vi "Export from Listbox to CSV.vi"(8 "error in (no error)":errorcluster, 10 "Name":string, 11 "MulticolumnListbox in":refnum<vi>) -> (0 "error out":errorcluster)   [LabVIEW 2019, in "Control Addon System Explorer.lvlib"]
uses:
  Control Addon System Explorer.lvlib
  Addon Shared/Control Addon Shared.lvlib
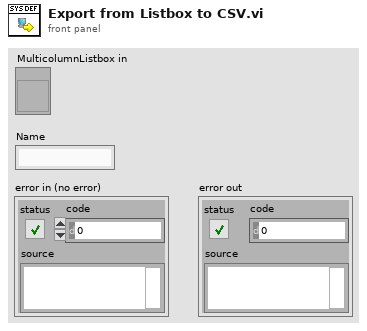
[diagram p1: front panel]
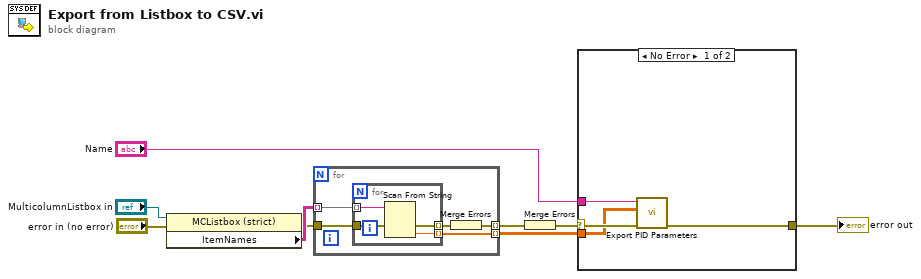
[diagram p0: block diagram]
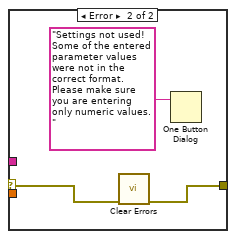
[diagram p2: hidden frame]
diagram:
  n1 = property class="MCListbox (strict)"(reference="MulticolumnListbox in", error in="error in (no error)") -> (error out=w5:errorcluster, "ItemNames"=w6:string[][])  [unwired: 1 out]
  n2 = for {
    tunnel: w6 -> [w14] mode=indexing
    tunnel: [w13] -> w1 mode=indexing
    tunnel: [w12] -> w9 mode=indexing
    tunnel: w5 -> [w10]
    n3 = for {
      tunnel: w14 -> [w18] mode=indexing
      tunnel: [w17] -> w13 mode=indexing
      tunnel: [w16] -> w11 mode=indexing
      tunnel: w10 -> [w15]
      n4 = Scan From String(input string=w18, error in=w15) -> (error out=w16:errorcluster, output 1=w17:dbl)  [unwired: 3 in, 2 out]
    }
    n5 = Merge Errors(w11) -> (w12:errorcluster)
  }
  n6 = Merge Errors(w9) -> (w4:errorcluster)
  n7 = case shown="No Error" w4 {
    selector: w4 -> [w22 w25]
    tunnel: [w21 w23] -> w3
    tunnel: "Name" -> [w20 _]
    tunnel: w1 -> [w19 _]
    frame No Error {
      n8 = call "Export PID Parameters.vi"("error in"=w22, "Parameters"=w19, "Control Loop"=w20) -> ("error out"=w21:errorcluster)  [unwired: 8 in]
    }
    frame Error {
      n9 = call <vilib>:"Clear Errors.vi"("error in (no error)"=w25) -> ("error out"=w23:errorcluster)  [unwired: 5 in, 1 out]
      n10 = One Button Dialog(message="Settings not used!  Some of the entered parameter values were not in the correct format.  Please make sure you are entering only numeric values.") -> ()  [unwired: 1 in, 1 out]
    }
  }
  "error out" <- w3
